vi "write_eu_to_db.vi"(0 "reference in":refnum<class "Sig_DO_Simple.lvclass">, 11 "error in (no error)":errorcluster) -> (4 "reference out":refnum<class "Sig_DO_Simple.lvclass">, 15 "error out":errorcluster)   [LabVIEW 2019]
uses:
  Proccess_class/Proccess.lvclass
  Sig_DO_Simple.lvclass
  Logger_class/Priority.ctl
  Logger_class/Logger.lvclass
  Logger_class/EventCode.ctl
  Logger_class/EventData.ctl
  D:/LabASF/LabASF/src/Proccess_class/Proccess.lvclass
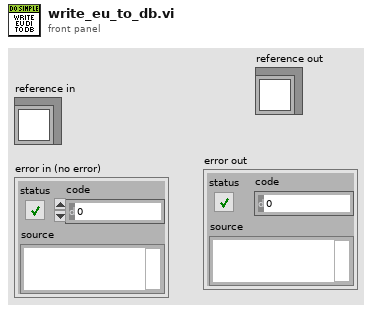
[diagram p1: front panel]
types:
  T1 = typedef "Sig_DO_Simple.lvclass/ObjectAttributes.ctl" = cluster{"DO":bool}
  T2 = typedef "Proccess.lvclass/ObjectAttributes.ctl" = cluster{"TagName":string, "ParentTagName":string, "MessageInterface":refnum<class "MessageInterface.lvclass">, "ConfigInterface":refnum<class "ConfigInterface.lvclass">, "Logger":refnum<class "Logger.lvclass">}
  T3 = typedef "Logger.lvclass/Priority.ctl" = enum16{"Alert", "Critical", "Error", "Warning", "Notice", "Informational", "Debug"}
  T4 = typedef "Logger.lvclass/EventCode.ctl" = enum16{"DI_EU_LO", "DI_EU_HI", "DIO_LO", "DIO_HI", "DI_RAW_LO", "DI_RAW_HI", "DO_LO", "DO_HI", "DA_OK", "DA_ALARM", "AA_HI", "AA_HIHI", "AA_LO", "AA_LOLO", "AA_OK", "CMD", "OUT_OF_RANGE_OK", "OUT_OF_RANGE_LO", "OUT_OF_RANGE_HI", "CONFIG", "DI_LO", "DI_HI"}
  T5 = typedef "Logger.lvclass/EventData.ctl" = cluster{"obj_tag":string, "event_tag":string, "code":T4, "Priority":T3, "Value":dbl, "Description":string, "Time Stamp":timestamp}
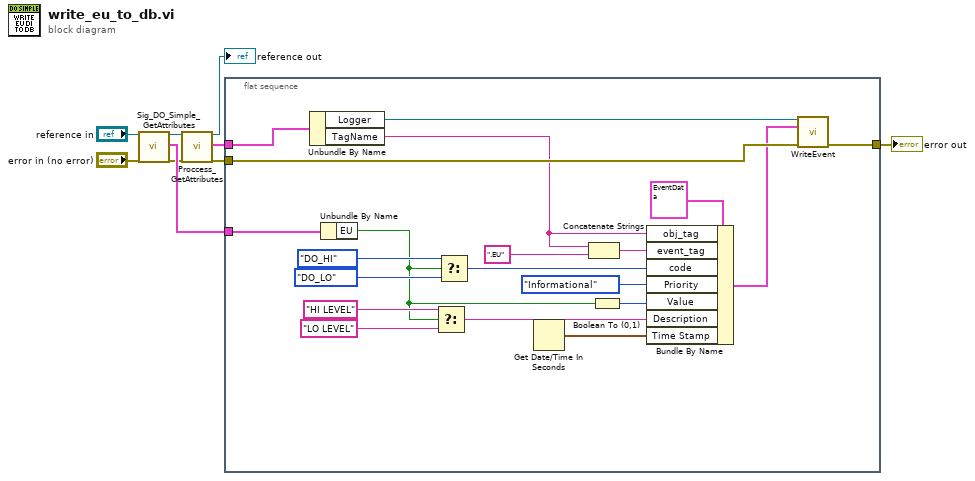
[diagram p0: block diagram]
diagram:
  n1 = call "Sig_DO_Simple_GetAttributes.vi"("reference in"="reference in", "error in (no error)"="error in (no error)") -> ("reference out"=w4:refnum<class "Sig_DO_Simple.lvclass">, "attributes"=w6:T1, "error out"=w5:errorcluster)  [unwired: 14 in, 1 out]
  n2 = call "Proccess_GetAttributes.vi"("reference in"=w4, "error in (no error)"=w5) -> ("reference out"=→"reference out":refnum<class "Sig_DO_Simple.lvclass">, "attributes"=w3:T2, "error out"=w7:errorcluster)  [unwired: 14 in, 1 out]
  n3 = flat-sequence {
    tunnel: w7 -> [w17]
    tunnel: w6 -> [w28]
    tunnel: w3 -> [w29]
    tunnel: [w11] -> w2
    frame #0 {
      n4 = Unbundle By Name(w29) -> ("Logger"=w27:refnum<class "Logger.lvclass">, "TagName"=w10:string)
      n5 = Unbundle By Name(w28) -> ("EU"=w14:bool)
      n6 = Select(t="HI LEVEL" ("Description"), s=w14, f="LO LEVEL" ("Description")) -> (s? t:f=w13:string)
      n7 = Select(t=EventCode."DO_HI" ("code"), s=w14, f=EventCode."DO_LO" ("code")) -> (s? t:f=w21:T4)
      n8 = Get Date/Time In Seconds() -> (seconds since 1Jan1904=w18:timestamp)
      n9 = Concatenate Strings(w10, ".EU" ("string")) -> (w24:string)
      n10 = Boolean To (0,1)(Boolean=w14) -> (0, 1=w19:i16)
      n11 = Bundle By Name(cluster=T5 {"obj_tag"="", "event_tag"="", "code"=enum."DI_RAW_LO", "Priority"=enum."Alert", "Value"=0.0, "Description"="", "Time Stamp"=timestamp(0 s since 1904-01-01)} ("Event"), "obj_tag"=w10, "event_tag"=w24, "code"=w21, "Priority"=Priority."Informational", "Value"=w19, "Description"=w13, "Time Stamp"=w18) -> (w12:T5)
      n12 = call "WriteEvent.vi"("reference in"=w27, "Event"=w12, "error in (no error)"=w17) -> ("error out"=w11:errorcluster)  [unwired: 11 in, 1 out]
    }
  }
  "error out" <- w2
